vi "RFSW Get SN State.vi"(8 "error in (no error)":errorcluster, 10 "SN":string) -> (0 "error out":errorcluster, 1 "PortAB_Array":i32[](array[numeric]), 2 "Connected?":bool, 3 "Ref_out":refnum<k24>, 4 "Model Name":string)   [LabVIEW 2020]
uses:
  C:/Projects/Github/LabVIEW-Tools/Mini-Circuits-RF-Switch/DLL/mcl_RF_Switch_Controller64.dll
  DLL/mcl_RF_Switch_Controller64.dll
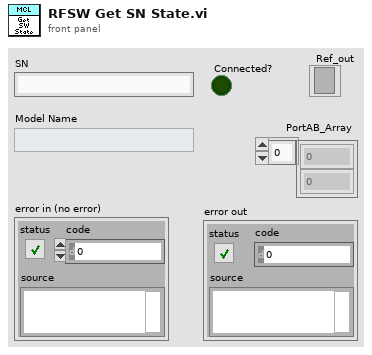
[diagram p1: front panel]
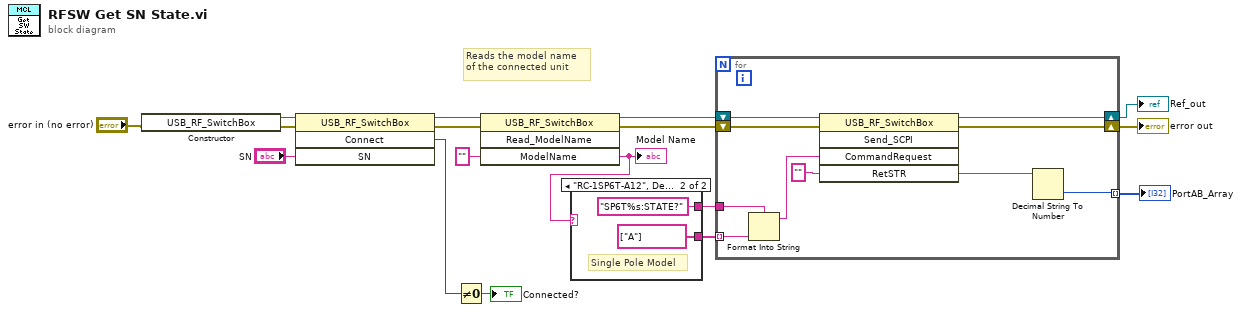
[diagram p0: block diagram]
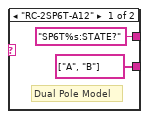
[diagram p2: hidden frame]
diagram:
  # "Reads the model name of the connected unit"
  n1 = constructor class="USB_RF_SwitchBox"(error in="error in (no error)") -> (reference out=w2:refnum<k24>, error out=w3:errorcluster)  [unwired: 2 in, 1 out]
  n2 = invoke class="USB_RF_SwitchBox" method="Connect"(reference=w2, error in=w3, "SN"="SN") -> (reference out=w15:refnum<k24>, error out=w14:errorcluster, "Connect"=w13:i32)  [unwired: 1 in, 1 out]
  n3 = Not Equal To 0?(x=w13) -> (x != 0?=→"Connected?":bool)
  n4 = invoke class="USB_RF_SwitchBox" method="Read_ModelName"(reference=w15, error in=w14, "ModelName"="") -> (reference out=w8:refnum<k24>, error out=w7:errorcluster, "ModelName"=w1:string)  [unwired: 1 in, 1 out]
  "Model Name" <- w1
  n5 = case shown="\"RC-1SP6T-A12\", Default" w1 {
    tunnel: ["SP6T%s:STATE?" "SP6T%s:STATE?"] -> w11
    tunnel: [string[] ["A", "B"] string[] ["A"]] -> w10
    frame "RC-2SP6T-A12" {
      # "Dual Pole Model"
    }
    frame "RC-1SP6T-A12", Default {
      # "Single Pole Model"
    }
  }
  n6 = for {
    shift-right: [w29] -> w16
    shift-left: w8 -> [w30]
    shift-right: [w28] -> w17
    shift-left: w7 -> [w31]
    tunnel: w10 -> [w27] mode=indexing
    tunnel: w11 -> [w24]
    tunnel: [w22] -> w6 mode=indexing
    n7 = Format Into String(format string=w24, w27) -> (resulting string=w26:string)  [unwired: 2 in, 1 out]
    n8 = invoke class="USB_RF_SwitchBox" method="Send_SCPI"(reference=w30, error in=w31, "CommandRequest"=w26, "RetSTR"="") -> (reference out=w29:refnum<k24>, error out=w28:errorcluster, "RetSTR"=w23:string)  [unwired: 1 in, 2 out]
    n9 = Decimal String To Number(string=w23) -> (number=w22:i32)  [unwired: 2 in, 1 out]
  }
  "error out" <- w17
  "Ref_out" <- w16
  "PortAB_Array" <- w6
